vi "ShowViewer.vi"(8 "error in (no error)":errorcluster, 11 "ViewerManager in":refnum<class "ViewerManager.lvclass">) -> (0 "error out":errorcluster, 3 "ViewerManager out":refnum<class "ViewerManager.lvclass">)   [LabVIEW 2019, in "ViewerManager.lvlib" / "ViewerManager.lvclass"]
uses:
  ViewerManager.lvclass
  C:/Program Files (x86)/National Instruments/LabVIEW 2019/vi.lib/ActorFramework/Actor/Actor.lvclass
  ResultsViewer/ResultsViewer/ResultsViewer.lvclass
  ViewerManager.lvclass/ViewerManager.ctl
  <vilib>/ActorFramework/Actor/Actor.lvclass
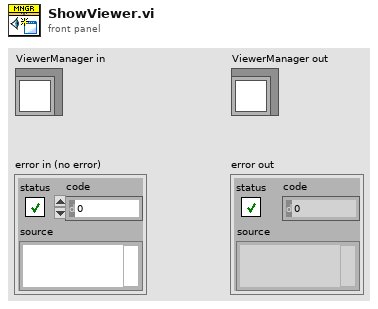
[diagram p1: front panel]
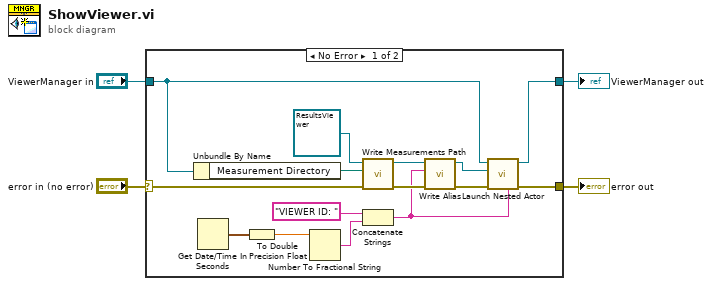
[diagram p0: block diagram]
diagram:
  n1 = case shown="No Error" "error in (no error)" {
    selector: "error in (no error)" -> [w19 w21]
    tunnel: [w18 w21] -> w3
    tunnel: [w8 w20] -> w1
    tunnel: "ViewerManager in" -> [w10 w20]
    frame No Error {
      n2 = Unbundle By Name(w10) -> ("Measurement Directory"=w9:path)
      n3 = Get Date/Time In Seconds() -> (seconds since 1Jan1904=w17:timestamp)
      n4 = To Double Precision Float(number=w17) -> (double precision float=w16:dbl)
      n5 = Number To Fractional String(number=w16) -> (F-format string=w6:string)  [unwired: 3 in]
      n6 = call-dynamic "Write Measurements Path.vi"("error in (no error)"=w19, "Measurements Path"=w9, "ResultsViewer in"=refnum<class "ResultsViewer.lvclass"> refnum ("ResultsViewer.lvlib:ResultsViewer.lvclass")) -> ("error out"=w13:errorcluster, "ResultsViewer out"=w11:refnum<class "ResultsViewer.lvclass">)  [unwired: 7 in]
      n7 = Concatenate Strings("VIEWER ID: " ("F-format string"), w6) -> (w5:string)
      n8 = call-dynamic "Write Alias.vi"("error in (no error)"=w13, "Alias"=w5, "ResultsViewer in"=w11) -> ("error out"=w15:errorcluster, "ResultsViewer out"=w14:refnum<class "ResultsViewer.lvclass">)  [unwired: 7 in]
      n9 = call <vilib>:"Launch Nested Actor.vi"("Debug Alias"=w5, "error in (no error)"=w15, "Nested Actor"=w14, "Caller Actor in"=w10) -> ("error out"=w18:errorcluster, "Caller Actor out"=w8:refnum<class "ViewerManager.lvclass">)  [unwired: 5 in, 1 out]
    }
    frame Error {
    }
  }
  "error out" <- w3
  "ViewerManager out" <- w1
